vi "WrtLog.vi"(8 "error in (no error)":errorcluster) -> (0 "error out":errorcluster)   [LabVIEW 2014]
uses:
  <vilib>/Utility/file.llb/Write To Spreadsheet File (string).vi
  Time/Time.lvlib
panel:
  in  "Duration[S]":dbl
  in  "WateringLog":path
  in  "No":u8
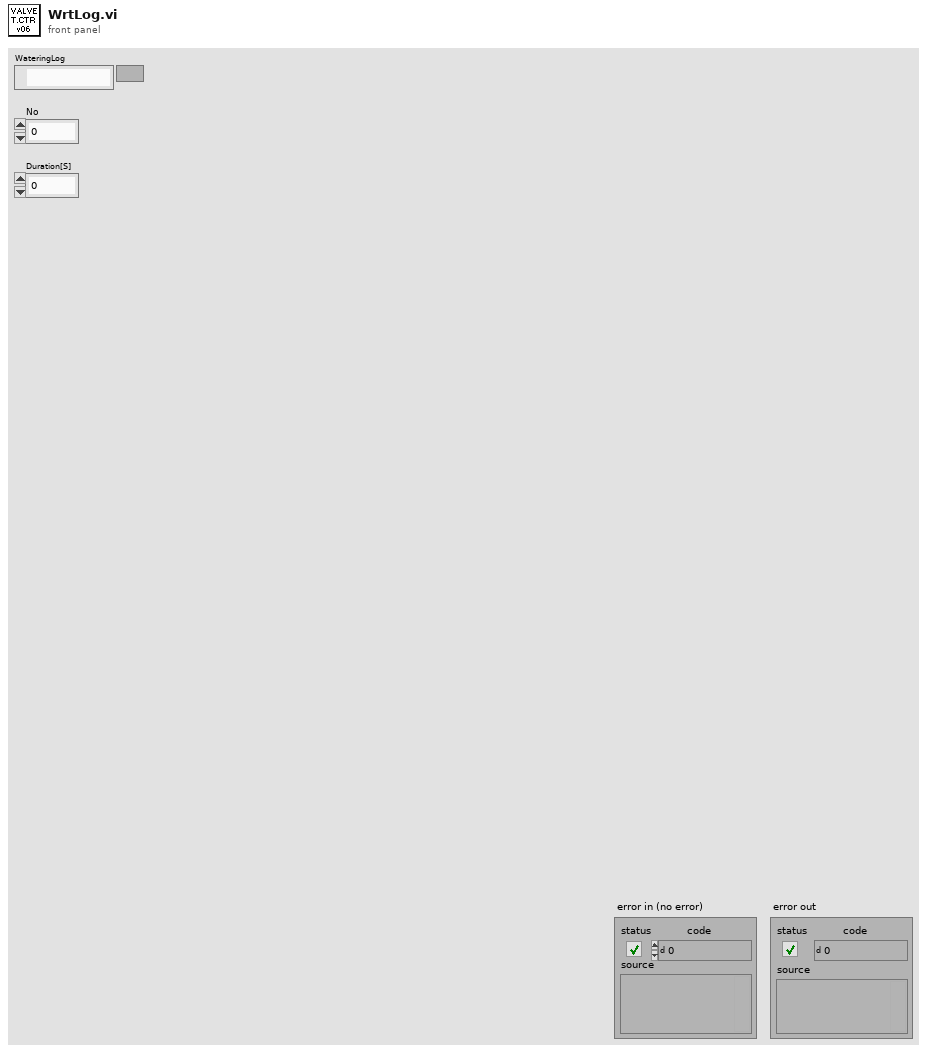
[diagram p1: front panel]
types:
  T1 = typedef "Time.lvlib/Local_DateTime_String.ctl" = cluster{"Local Date Time":string, "Local Date":string, "Local Time":string}
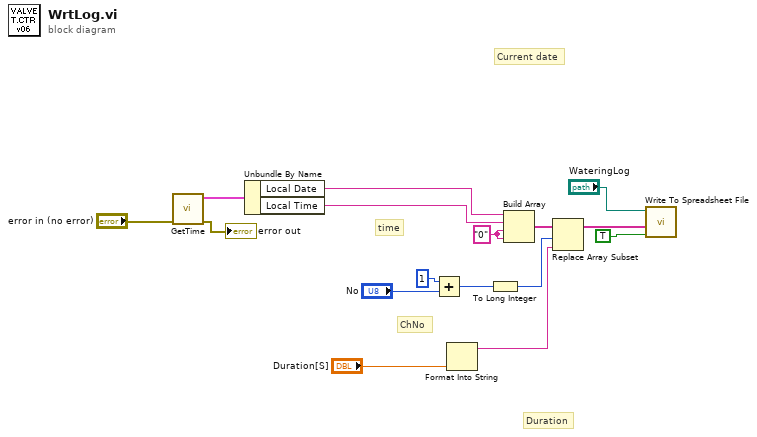
[diagram p0: block diagram]
diagram:
  w16 = "0" ("element")
  # "Current date"
  # "Duration"
  # "time"
  # "ChNo"
  n1 = call "GetTime.vi"("error in"="error in (no error)") -> ("error out"=→"error out":errorcluster, "Local Data/Time[String]"=w5:T1)  [unwired: 7 in, 2 out]
  n2 = Unbundle By Name(w5) -> ("Local Date"=w4:string, "Local Time"=w3:string)
  n3 = Add(x=u8 1, y="No") -> (x+y=w10:u8)
  n4 = Format Into String("Duration[S]") -> (resulting string=w6:string)  [unwired: 3 in, 1 out]
  n5 = To Long Integer(number=w10) -> (32bit integer=w12:i32)
  n6 = Build Array(w4, w3, w16, w16) -> (w11:string[])
  n7 = Replace Array Subset(array=w11, new element=w6, index=w12) -> (w15:string[])
  n8 = call-poly <vilib>:"Write To Spreadsheet File.vi"("append to file? (new file:F)"=TRUE, "1D data"=w15, "file path (dialog if empty)"="WateringLog") -> ()  [unwired: 5 in, 1 out]
